vi "_RT_CtrlLoop_D999_Process.vi"(6 "ExpVar in":refnum<class "ExpVar.lvclass">, 8 "error in (no error)":errorcluster, 11 "RS232ComPort in":refnum<class "RS232ComPort.lvclass">) -> ()   [LabVIEW 2018]
uses:
  PublicSubVI/NewExpVar/ExpVar.lvclass
  PublicSubVI/RS232/RS232ComPort.lvclass
  PublicSubVI/Ctl/_ctl_RT_D999_Command.ctl
  PublicSubVI/Ctl/_ctl_RT_SysLog.ctl
  PublicSubVI/Ctl/_ctl_RT_D999_Format.ctl
  PublicSubVI/Ctl/_ctl_RT_D999_Param.ctl
  PublicSubVI/Ctl/_ctl_RT_D999_Settings.ctl
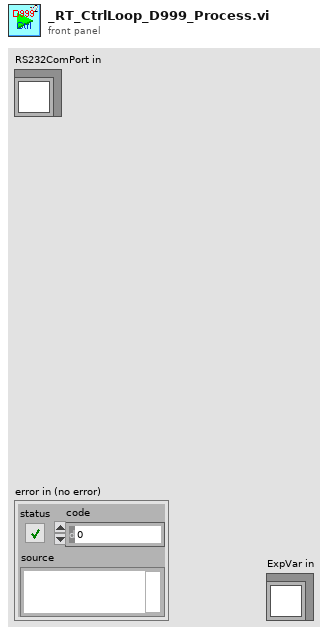
[diagram p1: front panel]
types:
  T1 = typedef "_ctl_RT_D999_Command.ctl" = cluster{"label":string, "value":variant}
  T2 = typedef "_ctl_RT_SysLog.ctl" = enum16{"None", "Initialize", "StartupRT", "StartupFPGA", "StartupAllocator", "GetMass", "SetWfmCode", "SetLaserCtrl", "SetTurboCtrl", "SetD999Ctrl", "Reconnecting...", "Interrupt", "StopRT"}
  T3 = typedef "_ctl_RT_D999_Format.ctl" = cluster{"Port":string, "Label":string, "Value":dbl}[]
  T4 = typedef "_ctl_RT_D999_Param.ctl" = cluster{"Enable":bool, "AI":cluster{"Label":string, "MultiValue":dbl, "AddValue":dbl}[], "AO":i16[], "Switch":bool[]}
  T5 = typedef "_ctl_RT_D999_Settings.ctl" = cluster{"Cmd":enum16{"None", "Init", "Write", "WriteAll", "Read", "ReadAll", "SetEnable", "SetParam", "ReadAO", "ReadSwitch", "ReportID"}, "Variant":variant}
  T6 = enum16{"None", "D999", "ExtAO", "ExtDO", "ExtDI_Label"}
  T7 = enum16{"None", "D999", "ExtAO", "ExtDO", "ExtDI_Label", "Signal_Remarks", "Script"}
  T8 = enum16{"via string label", "Laser", "Pressure", "TMP", "Script", "Signal Remarks", "ExtAO", "ExtDO", "ExtDI", "D999"}
  T9 = typedef "Semaphore RefNum" = refnum<k1>
  T10 = cluster{"Response Str":string, "VISA resource":refnum<visa-resource-name>, "DeviceExist?":bool, "semaphore":T9}
  T11 = cluster{"Label":string, "MultiValue":dbl, "AddValue":dbl}[]
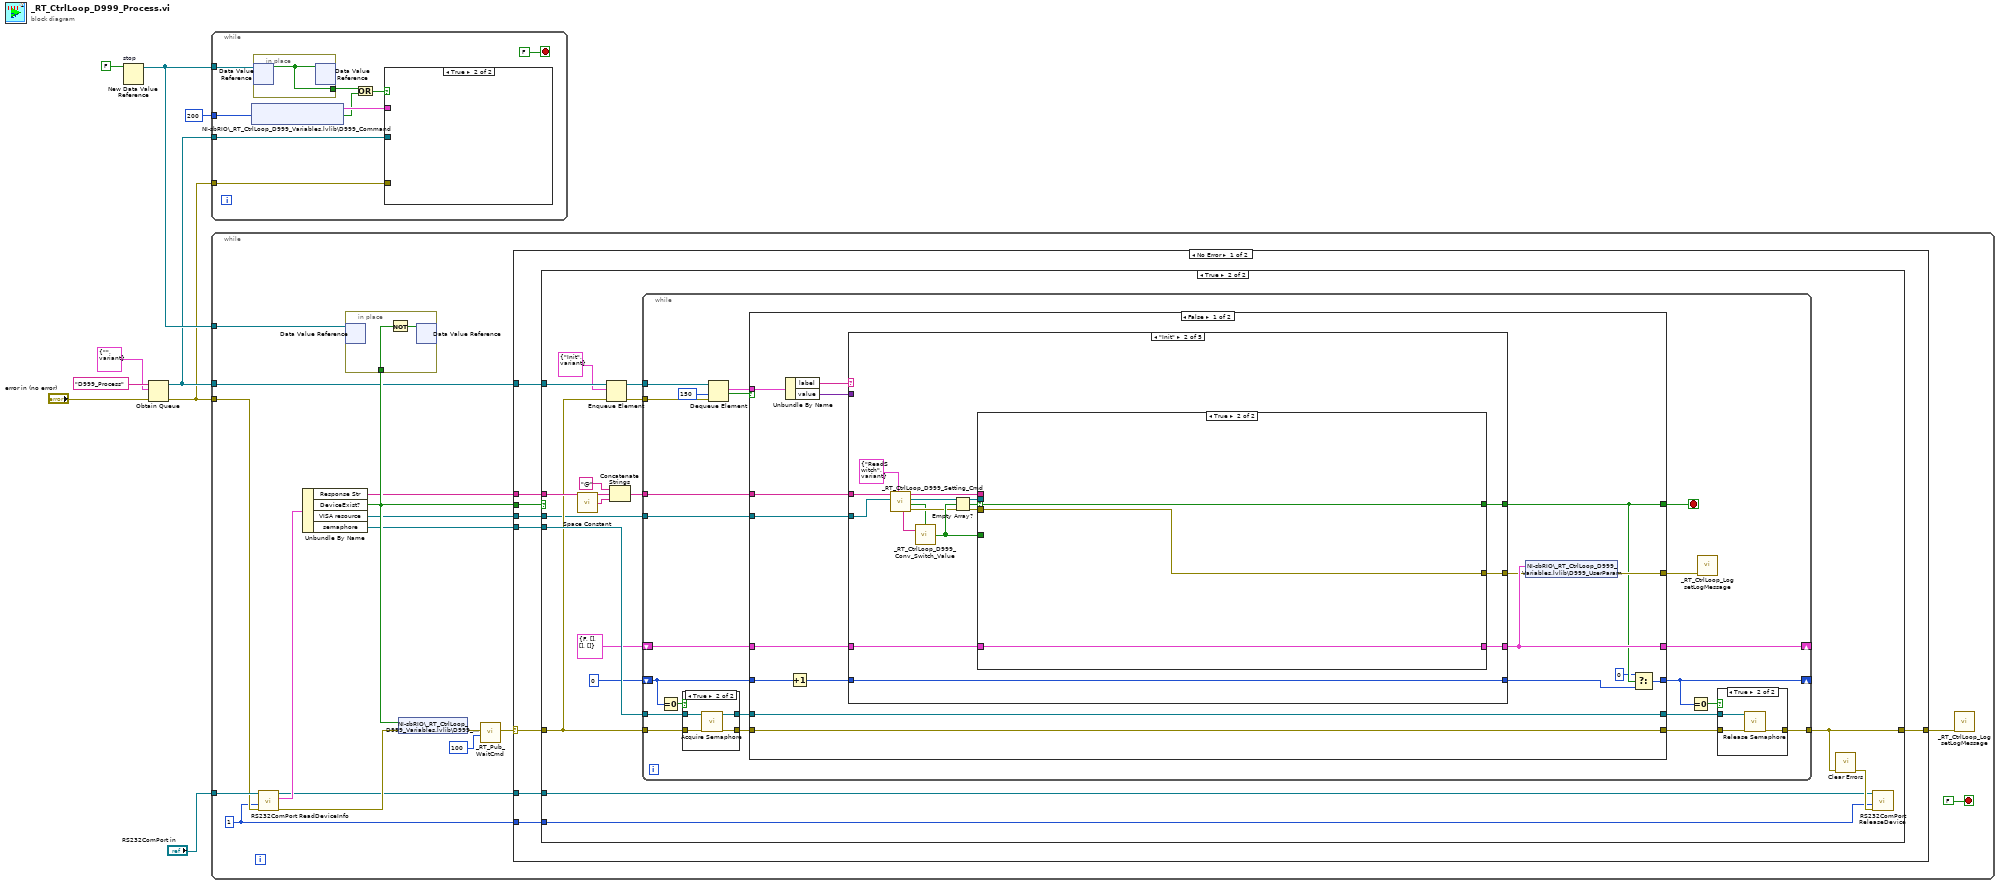
[diagram p0: block diagram]
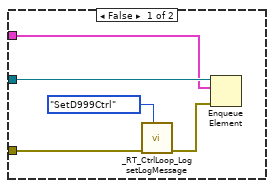
[diagram p2: hidden frame]
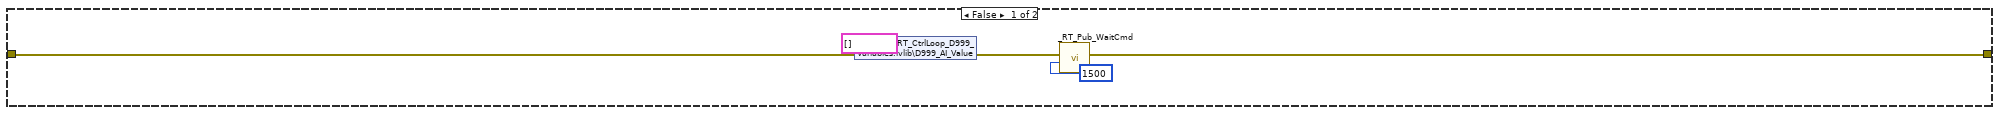
[diagram p3: hidden frame]
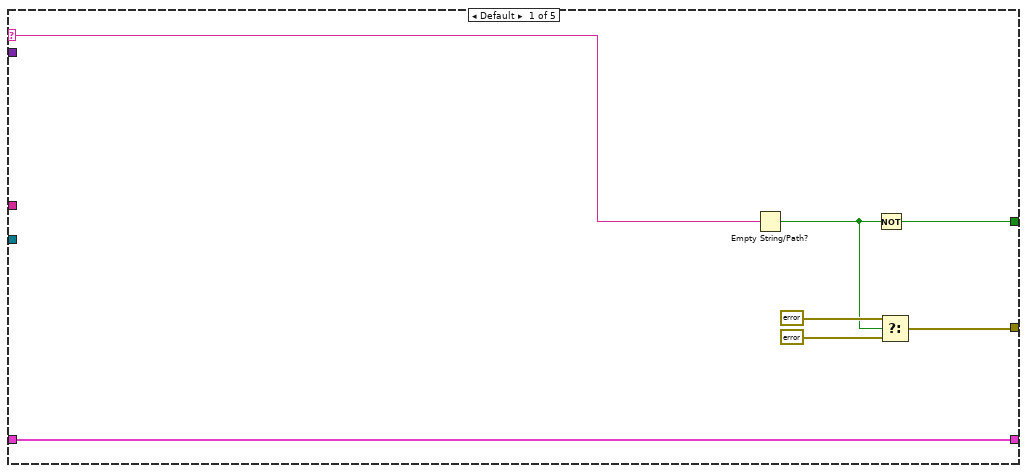
[diagram p6: hidden frame]
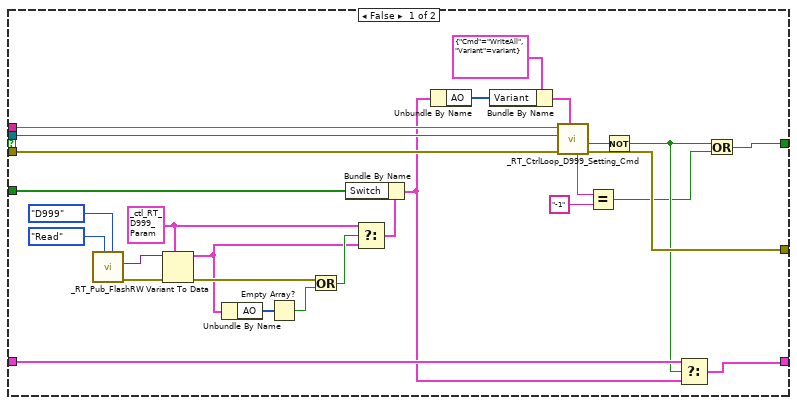
[diagram p7: hidden frame]
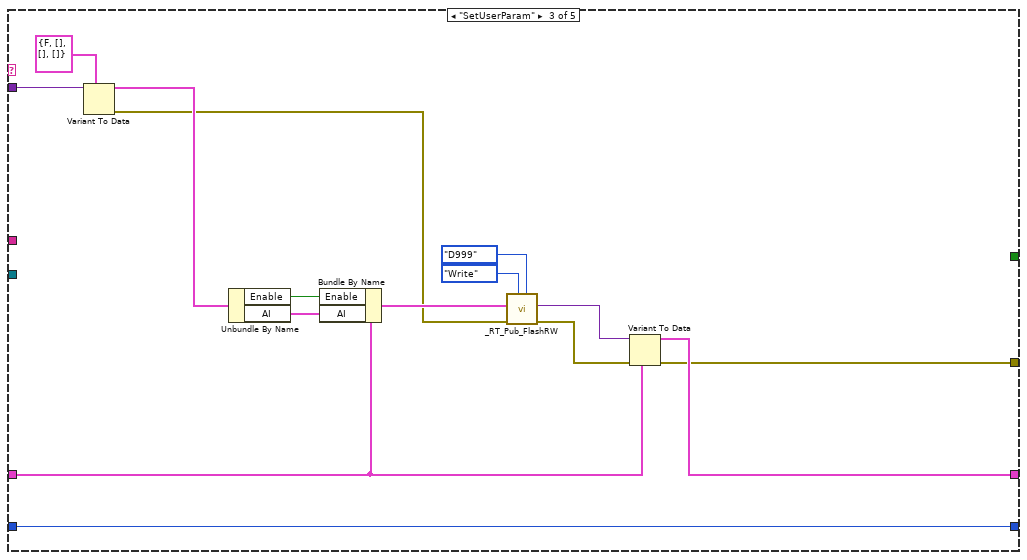
[diagram p8: hidden frame]
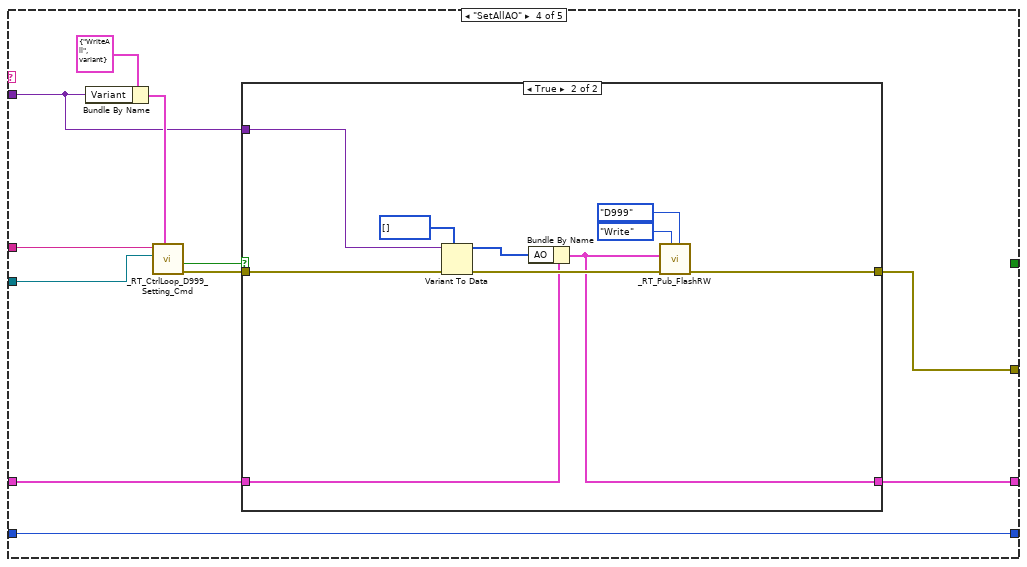
[diagram p9: hidden frame]
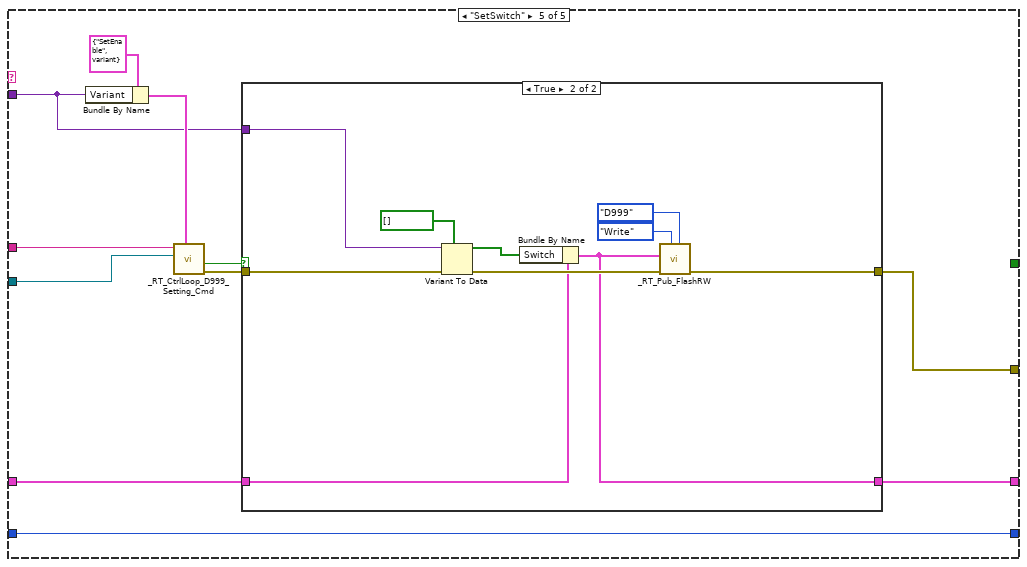
[diagram p11: hidden frame]
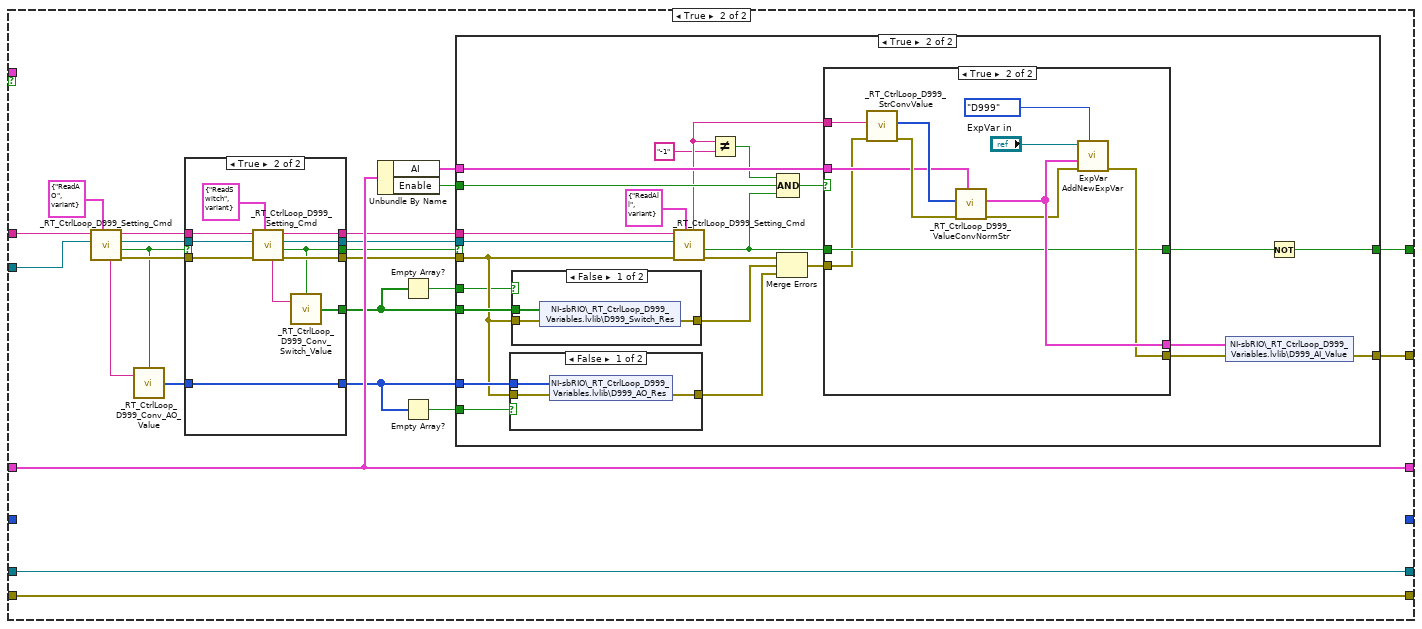
[diagram p13: hidden frame]
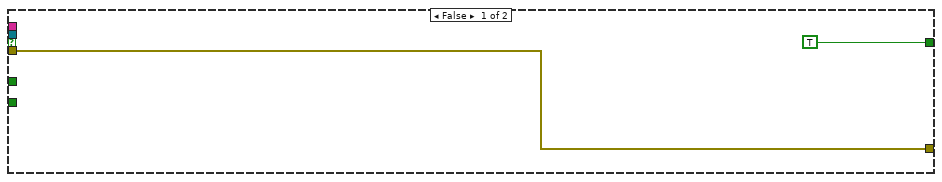
[diagram p14: hidden frame]
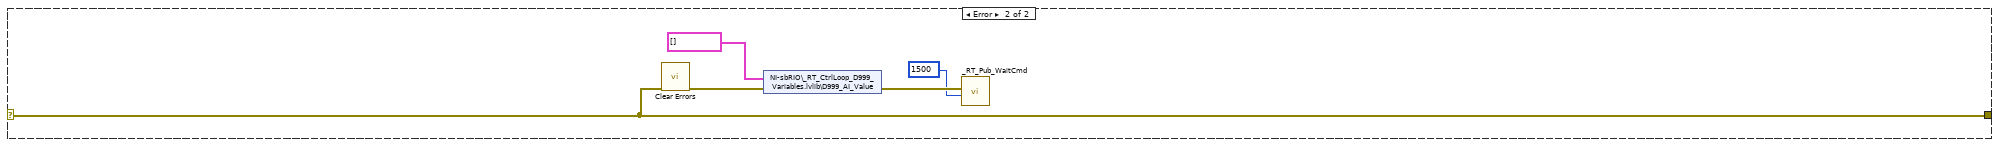
[diagram p19: hidden frame]
diagram:
  n1 = New Data Value Reference "stop"(data value=FALSE) -> (data value reference=w7:refnum<data-value>)  [unwired: 1 in, 1 out]
  n2 = Obtain Queue(name (unnamed)="D999_Process", element data type=T1 {"label"="", "value"=variant}, error in (no error)="error in (no error)") -> (queue out=w4:refnum<queue>, error out=w3:errorcluster)  [unwired: 2 in, 1 out]
  n3 = while {
    tunnel: w7 -> [w18]
    tunnel: w4 -> [w14]
    tunnel: w3 -> [w13]
    tunnel: 200 -> [w10]
    stop <- FALSE stop-if-true
    n4 = shared-variable "NI-sbRIO\\_RT_CtrlLoop_D999_Variables.lvlib\\D999_Command"(w10) -> (w12:T1, w11:bool)  [unwired: 1 in, 1 out]
    n5 = in-place {
      in-place-border: [w24] -> w15
      n6 = in-place-dvr #1(w18) -> (w24:bool)  [unwired: 1 out]
      n7 = in-place-dvr #1(w24) -> ()  [unwired: 2 out]
    }
    n8 = Or(x=w15, y=w11) -> (x .or. y?=w16:bool)
    n9 = case shown="True" w16 {
      tunnel: w12 -> [w20 _]
      tunnel: w14 -> [w22 _]
      tunnel: w13 -> [w21 _]
      frame False {
        n10 = call "_RT_CtrlLoop_Log setLogMessage.vi"("system type"=_ctl_RT_SysLog."SetD999Ctrl", "error in"=w21) -> ("error out"=w23:errorcluster)  [unwired: 8 in, 1 out]
        n11 = Enqueue Element(queue=w22, element=w20, error in (no error)=w23) -> ()  [unwired: 1 in, 3 out]
      }
      frame True {
      }
    }
  }
  n12 = while {
    tunnel: "RS232ComPort in" -> [w41]
    tunnel: w7 -> [w39]
    tunnel: w4 -> [w32]
    tunnel: w3 -> [w33]
    stop <- FALSE stop-if-true
    w25 = 1 ("DeviceIndex")
    n13 = call-dynamic "RS232ComPort ReadDeviceInfo.vi"("error in (no error)"=w33, "DeviceIndex"=w25, "RS232ComPort in"=w41) -> ("error out"=w37:errorcluster, "DeviceInfo"=w40:T10, "RS232ComPort out"=w26:refnum<class "RS232ComPort.lvclass">)  [unwired: 6 in]
    n14 = Unbundle By Name(w40) -> ("Response Str"=w31:string, "DeviceExist?"=w38:bool, "VISA resource"=w30:refnum<visa-resource-name>, "semaphore"=w29:T9)
    n15 = in-place {
      in-place-border: w38 -> [w329]
      n16 = in-place-dvr #2(w39) -> ()  [unwired: 2 out]
      n17 = Not(x=w329) -> (.not. x?=w328:bool)
      n18 = in-place-dvr #2(w328) -> ()  [unwired: 2 out]
    }
    n19 = shared-variable "NI-sbRIO\\_RT_CtrlLoop_D999_Variables.lvlib\\D999_Exist"(w38, error in=w37) -> (error out=w36:errorcluster)
    n20 = call "_RT_Pub_WaitCmd.vi"("milliseconds to wait"=u32 100, "error in (no error)"=w36) -> ("error out"=w34:errorcluster)  [unwired: 9 in]
    n21 = case shown="No Error" w34 {
      selector: w34 -> [w49 w325]
      tunnel: w38 -> [w50 _]
      tunnel: w32 -> [w48 _]
      tunnel: w31 -> [w47 _]
      tunnel: w30 -> [w46 _]
      tunnel: w29 -> [w45 _]
      tunnel: [w44 w325] -> w28
      tunnel: w26 -> [w43 _]
      tunnel: w25 -> [w42 _]
      frame No Error {
        n22 = case shown="True" w50 {
          tunnel: w49 -> [w54 w63]
          tunnel: w48 -> [_ w66]
          tunnel: w47 -> [_ w70]
          tunnel: w46 -> [_ w60]
          tunnel: w45 -> [_ w64]
          tunnel: [w51 w65] -> w44
          tunnel: w43 -> [_ w68]
          tunnel: w42 -> [_ w67]
          frame False {
            n23 = shared-variable "NI-sbRIO\\_RT_CtrlLoop_D999_Variables.lvlib\\D999_AI_Value"(T3 [] ("D999_AI_Value"), error in=w54) -> (error out=w52:errorcluster)
            n24 = call "_RT_Pub_WaitCmd.vi"("milliseconds to wait"=u32 1500, "error in (no error)"=w52) -> ("error out"=w51:errorcluster)  [unwired: 9 in]
          }
          frame True {
            n25 = call <vilib>:"Space Constant.vi"() -> ("String"=w71:string)
            n26 = Enqueue Element(queue=w66, element=T1 {"label"="Init", "value"=variant}, error in (no error)=w63) -> (queue out=w62:refnum<queue>, error out=w61:errorcluster)  [unwired: 1 in, 1 out]
            n27 = Concatenate Strings("@" ("string"), w70, w71) -> (w59:string)
            n28 = while {
              tunnel: w62 -> [w93]
              tunnel: w61 -> [w92]
              shift-right: [w87] -> _
              shift-left: T4 {"Enable"=FALSE, "AI"=[], "AO"=[], "Switch"=[]} ("D999_Param") -> [w88]
              tunnel: [w77] -> w65
              tunnel: w64 -> [w83]
              tunnel: w63 -> [w82]
              tunnel: w60 -> [w84]
              tunnel: w59 -> [w85]
              shift-right: [w74] -> _
              shift-left: 0 -> [w76]
              stop <- w89 stop-if-true
              n29 = Equal To 0?(x=w76) -> (x = 0?=w75:bool)
              n30 = case shown="True" w75 {
                tunnel: w83 -> [w100 w104]
                tunnel: w82 -> [w99 w103]
                tunnel: [w100 w102] -> w81
                tunnel: [w99 w101] -> w80
                frame False {
                }
                frame True {
                  n31 = call <vilib>:"Acquire Semaphore.vi"("error in (no error)"=w103, "semaphore"=w104) -> ("error out"=w101:errorcluster, "semaphore out"=w102:T9)  [unwired: 3 in, 1 out]
                }
              }
              n32 = Dequeue Element(queue=w93, timeout in ms (-1)=150, error in (no error)=w92) -> (element=w90:T1, timed out?=w91:bool)  [unwired: 2 out]
              n33 = case shown="False" w91 {
                tunnel: w90 -> [w121 _]
                tunnel: [w107 w247] -> w89
                tunnel: w88 -> [w118 w253]
                tunnel: [w115 w253] -> w87
                tunnel: [w113 w244] -> w86
                tunnel: w81 -> [w111 w243]
                tunnel: w80 -> [w112 w242]
                tunnel: [w112 w242] -> w78
                tunnel: w85 -> [w117 w246]
                tunnel: w84 -> [w116 w245]
                tunnel: [w111 w243] -> w79
                tunnel: w76 -> [w110 _]
                tunnel: [w108 _] -> w74
                frame False {
                  n34 = Unbundle By Name(w121) -> ("label"=w120:string, "value"=w119:variant)
                  n35 = Increment(x=w110) -> (x+1=w109:i32)
                  n36 = case shown="\"Init\"" w120 {
                    selector: w120 -> [w127 _ _ _ _]
                    tunnel: w119 -> [_ _ w189 w195 w218]
                    tunnel: [w122 w142 _ _ _] -> w107
                    tunnel: w118 -> [w128 w140 w186 w197 w220]
                    tunnel: [w128 w139 w185 w196 w219] -> w115
                    tunnel: [w124 w137 w184 w193 w216] -> w114
                    tunnel: w117 -> [_ w132 _ w192 w215]
                    tunnel: w116 -> [_ w131 _ w191 w214]
                    tunnel: [_ w136 w183 w190 w213] -> w106
                    tunnel: w109 -> [_ w136 w183 w190 w213]
                    frame Default {
                      n37 = Empty String/Path?(string/path=w127) -> (empty?=w123:bool)
                      n38 = Not(x=w123) -> (.not. x?=w122:bool)
                      n39 = Select(t=errorcluster {"status"=FALSE, "code"=0, "source"=""}, s=w123, f=errorcluster {"status"=TRUE, "code"=6001, "source"="unknown command"} ("error out")) -> (s? t:f=w124:errorcluster)
                    }
                    frame "Init" {
                      n40 = call "_RT_CtrlLoop_D999_Setting_Cmd.vi"("CmdParam"=T5 {"Cmd"=enum."ReadSwitch", "Variant"=variant}, "VISA resource In"=w131, "headcmd in"=w132) -> ("error out"=w138:errorcluster, "valid"=w134:bool, "VISA resource Out"=w129:refnum<visa-resource-name>, "headcmd out"=w130:string, "Response Str"=w133:string)  [unwired: 4 in]
                      n41 = call "_RT_CtrlLoop_D999_Conv_Switch_Value.vi"("valid"=w134, "Response Str"=w133) -> ("switch array"=w141:bool[])  [unwired: 1 in]
                      n42 = Empty Array?(array=w141) -> (empty?=w143:bool)
                      n43 = case shown="True" w143 {
                        selector: w143 -> [_ w174]
                        tunnel: [w148 w174] -> w142
                        tunnel: w141 -> [w166 _]
                        tunnel: w140 -> [w165 w173]
                        tunnel: [w164 w173] -> w139
                        tunnel: w138 -> [w163 w172]
                        tunnel: [w162 w172] -> w137
                        tunnel: w130 -> [w158 _]
                        tunnel: w129 -> [w157 _]
                        frame False {
                          w169 = T4 {"Enable"=FALSE, "AI"=[{"Label"="", "MultiValue"=1.0, "AddValue"=0.0}, {"Label"="", "MultiValue"=1.0, "AddValue"=0.0}, {"Label"="", "MultiValue"=1.0, "AddValue"=0.0}, {"Label"="", "MultiValue"=1.0, "AddValue"=0.0}, {"Label"="", "MultiValue"=1.0, "AddValue"=0.0}, {"Label"="", "MultiValue"=1.0, "AddValue"=0.0}, {"Label"="", "MultiValue"=1.0, "AddValue"=0.0}, {"Label"="", "MultiValue"=1.0, "AddValue"=0.0}, {"Label"="", "MultiValue"=1.0, "AddValue"=0.0}, {"Label"="", "MultiValue"=1.0, "AddValue"=0.0}, {"Label"="", "MultiValue"=1.0, "AddValue"=0.0}, {"Label"="", "MultiValue"=1.0, "AddValue"=0.0}], "AO"=[0, 0, 0, 0, 0, 0, 0, 0, 0], "Switch"=[FALSE, FALSE, FALSE, FALSE]} ("D999_Param")
                          n44 = call "_RT_Pub_FlashRW.vi"("FileEnum"=T6."D999" ("FileName"), "State"=enum16{"Read", "Write"}."Read") -> ("error out"=w170:errorcluster, "Value"=w171:variant)  [unwired: 7 in, 1 out]
                          n45 = Variant To Data(error in=w170, type=w169, Variant=w171) -> (data=w149:T4, error out=w151:errorcluster)
                          n46 = Unbundle By Name(w149) -> ("AO"=w153:i16[])
                          n47 = Empty Array?(array=w153) -> (empty?=w150:bool)
                          n48 = Or(x=w151, y=w150) -> (x .or. y?=w152:bool)
                          n49 = Select(t=w169, s=w152, f=w149) -> (s? t:f=w156:T4)
                          n50 = Bundle By Name(cluster=w156, "Switch"=w166) -> (w155:T4)
                          n51 = Unbundle By Name(w155) -> ("AO"=w154:i16[])
                          n52 = Bundle By Name(cluster=T5 {"Cmd"=enum."WriteAll", "Variant"=variant} ("CmdParam"), "Variant"=w154) -> (w160:T5)
                          n53 = call "_RT_CtrlLoop_D999_Setting_Cmd.vi"("CmdParam"=w160, "error in (no error)"=w163, "VISA resource In"=w157, "headcmd in"=w158) -> ("error out"=w162:errorcluster, "valid"=w159:bool, "Response Str"=w147:string)  [unwired: 3 in, 2 out]
                          n54 = Equal?(x=w147, y="-1" ("x")) -> (x = y?=w144:bool)
                          n55 = Not(x=w159) -> (.not. x?=w146:bool)
                          n56 = Select(t=w165, s=w146, f=w155) -> (s? t:f=w164:T4)
                          n57 = Or(x=w146, y=w144) -> (x .or. y?=w148:bool)
                        }
                        frame True {
                        }
                      }
                    }
                    frame "SetUserParam" {
                      n58 = Variant To Data(type=T4 {"Enable"=FALSE, "AI"=[], "AO"=[], "Switch"=[]} ("D999_Param"), Variant=w189) -> (data=w187:T4, error out=w175:errorcluster)  [unwired: 1 in]
                      n59 = Unbundle By Name(w187) -> ("Enable"=w182:bool, "AI"=w181:T11)
                      n60 = Bundle By Name(cluster=w186, "Enable"=w182, "AI"=w181) -> (w178:T4)
                      n61 = call "_RT_Pub_FlashRW.vi"("FileEnum"=T7."D999", "State"=enum16{"Read", "Write"}."Write", "error in (no error)"=w175, "DataIn"=w178) -> ("error out"=w176:errorcluster, "Value"=w177:variant)  [unwired: 5 in, 1 out]
                      n62 = Variant To Data(error in=w176, type=w186, Variant=w177) -> (data=w185:T4, error out=w184:errorcluster)
                    }
                    frame "SetAllAO" {
                      n63 = Bundle By Name(cluster=T5 {"Cmd"=enum."WriteAll", "Variant"=variant} ("CmdParam"), "Variant"=w195) -> (w199:T5)
                      n64 = call "_RT_CtrlLoop_D999_Setting_Cmd.vi"("CmdParam"=w199, "VISA resource In"=w191, "headcmd in"=w192) -> ("error out"=w194:errorcluster, "valid"=w198:bool)  [unwired: 4 in, 3 out]
                      n65 = case shown="True" w198 {
                        tunnel: w197 -> [w202 w207]
                        tunnel: [w202 w206] -> w196
                        tunnel: w195 -> [_ w205]
                        tunnel: w194 -> [w201 w204]
                        tunnel: [w201 w203] -> w193
                        frame False {
                        }
                        frame True {
                          n66 = Variant To Data(error in=w204, type=i16[] [] ("AO"), Variant=w205) -> (data=w211:i16[], error out=w208:errorcluster)
                          n67 = Bundle By Name(cluster=w207, "AO"=w211) -> (w206:T4)
                          n68 = call "_RT_Pub_FlashRW.vi"("FileEnum"=T6."D999" ("FileName"), "State"=enum16{"Read", "Write"}."Write", "error in (no error)"=w208, "DataIn"=w206) -> ("error out"=w203:errorcluster)  [unwired: 5 in, 2 out]
                        }
                      }
                    }
                    frame "SetSwitch" {
                      n69 = Bundle By Name(cluster=T5 {"Cmd"=enum."SetEnable", "Variant"=variant} ("CmdParam"), "Variant"=w218) -> (w222:T5)
                      n70 = call "_RT_CtrlLoop_D999_Setting_Cmd.vi"("CmdParam"=w222, "VISA resource In"=w214, "headcmd in"=w215) -> ("error out"=w217:errorcluster, "valid"=w221:bool)  [unwired: 4 in, 3 out]
                      n71 = case shown="True" w221 {
                        tunnel: w220 -> [w225 w231]
                        tunnel: [w225 w230] -> w219
                        tunnel: w218 -> [_ w229]
                        tunnel: w217 -> [w224 w228]
                        tunnel: [w224 w227] -> w216
                        frame False {
                        }
                        frame True {
                          n72 = Variant To Data(error in=w228, type=bool[] [] ("AO"), Variant=w229) -> (data=w235:bool[], error out=w232:errorcluster)
                          n73 = Bundle By Name(cluster=w231, "Switch"=w235) -> (w230:T4)
                          n74 = call "_RT_Pub_FlashRW.vi"("FileEnum"=T6."D999" ("FileName"), "State"=enum16{"Read", "Write"}."Write", "error in (no error)"=w232, "DataIn"=w230) -> ("error out"=w227:errorcluster)  [unwired: 5 in, 2 out]
                        }
                      }
                    }
                  }
                  n75 = shared-variable "NI-sbRIO\\_RT_CtrlLoop_D999_Variables.lvlib\\D999_UserParam"(w115, error in=w114) -> (error out=w113:errorcluster)
                  n76 = Select(t=0, s=w107, f=w106) -> (s? t:f=w108:i32)
                }
                frame True {
                  n77 = call "_RT_CtrlLoop_D999_Setting_Cmd.vi"("CmdParam"=T5 {"Cmd"=enum."ReadAO", "Variant"=variant}, "VISA resource In"=w245, "headcmd in"=w246) -> ("error out"=w256:errorcluster, "valid"=w241:bool, "VISA resource Out"=w257:refnum<visa-resource-name>, "headcmd out"=w258:string, "Response Str"=w255:string)  [unwired: 4 in]
                  n78 = call "_RT_CtrlLoop_D999_Conv_AO_Value.vi"("valid"=w241, "Response Str"=w255) -> ("AO Array"=w254:i32[])  [unwired: 1 in]
                  n79 = case shown="True" w241 {
                    selector: w241 -> [w311 _]
                    tunnel: w258 -> [w309 w321]
                    tunnel: w257 -> [w308 w320]
                    tunnel: w256 -> [w310 w319]
                    tunnel: [w311 w312] -> w240
                    tunnel: [_ w317] -> w239
                    tunnel: [w310 w316] -> w250
                    tunnel: w254 -> [w307 w315]
                    tunnel: [w307 w315] -> w238
                    tunnel: [w309 w314] -> w252
                    tunnel: [w308 w313] -> w251
                    frame False {
                    }
                    frame True {
                      n80 = call "_RT_CtrlLoop_D999_Setting_Cmd.vi"("CmdParam"=T5 {"Cmd"=enum."ReadSwitch", "Variant"=variant}, "error in (no error)"=w319, "VISA resource In"=w320, "headcmd in"=w321) -> ("error out"=w316:errorcluster, "valid"=w312:bool, "VISA resource Out"=w313:refnum<visa-resource-name>, "headcmd out"=w314:string, "Response Str"=w318:string)  [unwired: 3 in]
                      n81 = call "_RT_CtrlLoop_D999_Conv_Switch_Value.vi"("valid"=w312, "Response Str"=w318) -> ("switch array"=w317:bool[])  [unwired: 1 in]
                    }
                  }
                  n82 = Unbundle By Name(w253) -> ("AI"=w248:T11, "Enable"=w249:bool)
                  n83 = Empty Array?(array=w239) -> (empty?=w237:bool)
                  n84 = Empty Array?(array=w238) -> (empty?=w236:bool)
                  n85 = case shown="True" w240 {
                    tunnel: w252 -> [_ w284]
                    tunnel: w251 -> [_ w283]
                    tunnel: w250 -> [w261 w269]
                    tunnel: w239 -> [_ w276]
                    tunnel: w238 -> [_ w275]
                    tunnel: w249 -> [_ w281]
                    tunnel: w248 -> [_ w280]
                    tunnel: [w261 w278] -> w244
                    tunnel: [TRUE w267] -> w247
                    tunnel: w237 -> [_ w265]
                    tunnel: w236 -> [_ w266]
                    frame False {
                    }
                    frame True {
                      n86 = case shown="False" w266 {
                        tunnel: w275 -> [w292 _]
                        tunnel: [w291 w293] -> w272
                        tunnel: w269 -> [w290 w293]
                        frame False {
                          n87 = shared-variable "NI-sbRIO\\_RT_CtrlLoop_D999_Variables.lvlib\\D999_AO_Res"(w292, error in=w290) -> (error out=w291:errorcluster)
                        }
                        frame True {
                        }
                      }
                      n88 = case shown="False" w265 {
                        tunnel: w276 -> [w288 _]
                        tunnel: [w287 w289] -> w273
                        tunnel: w269 -> [w286 w289]
                        frame False {
                          n89 = shared-variable "NI-sbRIO\\_RT_CtrlLoop_D999_Variables.lvlib\\D999_Switch_Res"(w288, error in=w286) -> (error out=w287:errorcluster)
                        }
                        frame True {
                        }
                      }
                      n90 = call "_RT_CtrlLoop_D999_Setting_Cmd.vi"("CmdParam"=T5 {"Cmd"=enum."ReadAll", "Variant"=variant}, "error in (no error)"=w269, "VISA resource In"=w283, "headcmd in"=w284) -> ("error out"=w274:errorcluster, "valid"=w270:bool, "Response Str"=w264:string)  [unwired: 3 in, 2 out]
                      n91 = Not Equal?(x=w264, y="-1") -> (x != y?=w262:bool)
                      n92 = Compound Arithmetic op=AND(w262, w281, w270) -> (w282:bool)
                      n93 = Merge Errors(w274, w273, w272) -> (w271:errorcluster)
                      n94 = case shown="True" w282 {
                        tunnel: [_ w303] -> w277
                        tunnel: w280 -> [_ w302]
                        tunnel: [w295 w300] -> w279
                        tunnel: w264 -> [_ w298]
                        tunnel: w271 -> [w295 w296]
                        tunnel: w270 -> [w294 w297]
                        tunnel: [w294 w297] -> w268
                        frame False {
                        }
                        frame True {
                          n95 = call "_RT_CtrlLoop_D999_StrConvValue.vi"("error in (no error)"=w296, "Response Str"=w298) -> ("error IO"=w305:errorcluster, "appended array"=w306:i32[])  [unwired: 8 in]
                          n96 = call "_RT_CtrlLoop_D999_ValueConvNormStr.vi"("AI_Param"=w302, "error in (no error)"=w305, "appended array"=w306) -> ("error out"=w301:errorcluster, "EC Format"=w303:T3)  [unwired: 7 in]
                          n97 = call-dynamic "ExpVar AddNewExpVar.vi"("VarType"=T8."D999", "error in (no error)"=w301, "Var"=w303, "ExpVar in"="ExpVar in") -> ("error out"=w300:errorcluster)  [unwired: 6 in, 1 out]
                        }
                      }
                      n98 = shared-variable "NI-sbRIO\\_RT_CtrlLoop_D999_Variables.lvlib\\D999_AI_Value"(w277, error in=w279) -> (error out=w278:errorcluster)
                      n99 = Not(x=w268) -> (.not. x?=w267:bool)
                    }
                  }
                }
              }
              n100 = Equal To 0?(x=w74) -> (x = 0?=w73:bool)
              n101 = call "_RT_CtrlLoop_Log setLogMessage.vi"("error in"=w86) -> ()  [unwired: 9 in, 2 out]
              n102 = case shown="True" w73 {
                tunnel: w79 -> [_ w98]
                tunnel: w78 -> [w95 w97]
                tunnel: [w95 w96] -> w77
                frame False {
                }
                frame True {
                  n103 = call <vilib>:"Release Semaphore.vi"("error in (no error)"=w97, "semaphore"=w98) -> ("error out"=w96:errorcluster)  [unwired: 4 in, 1 out]
                }
              }
            }
            n104 = call <vilib>:"Clear Errors.vi"("error in (no error)"=w65) -> ("error out"=w69:errorcluster)  [unwired: 5 in, 1 out]
            n105 = call "RS232ComPort ReleaseDevice.vi"("error in (no error)"=w69, "DeviceIndex"=w67, "RS232ComPort in"=w68) -> ()  [unwired: 8 in, 1 out]
          }
        }
      }
      frame Error {
        n106 = call <vilib>:"Clear Errors.vi"("error in (no error)"=w325) -> ("error out"=w324:errorcluster)  [unwired: 5 in, 1 out]
        n107 = shared-variable "NI-sbRIO\\_RT_CtrlLoop_D999_Variables.lvlib\\D999_AI_Value"(T3 [] ("D999_AI_Value"), error in=w324) -> (error out=w326:errorcluster)
        n108 = call "_RT_Pub_WaitCmd.vi"("milliseconds to wait"=u32 1500, "error in (no error)"=w326) -> ()  [unwired: 9 in, 1 out]
      }
    }
    n109 = call "_RT_CtrlLoop_Log setLogMessage.vi"("error in"=w28) -> ()  [unwired: 9 in, 2 out]
  }
